vi "IL Chain Handle Last Ack.vi"(8 "error in (no error)":errorcluster, 10 "Last Ack":refnum<class "Last Ack.lvclass">, 11 "Interlock Chain in":refnum<class "Interlock Chain.lvclass">) -> (0 "error out":errorcluster, 3 "Interlock Chain out":refnum<class "Interlock Chain.lvclass">)   [LabVIEW 2015, in "Interlocks.lvlib" / "Interlock Chain.lvclass"]
uses:
  Interlock Chain.lvclass
  <vilib>/ActorFramework/LastAck/Last Ack.lvclass
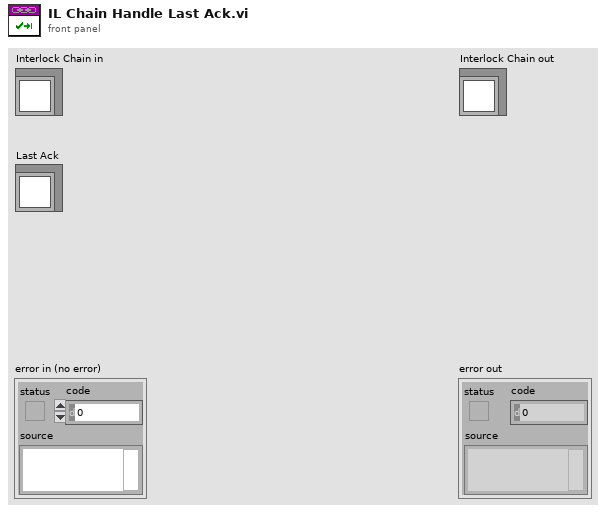
[diagram p1: front panel]
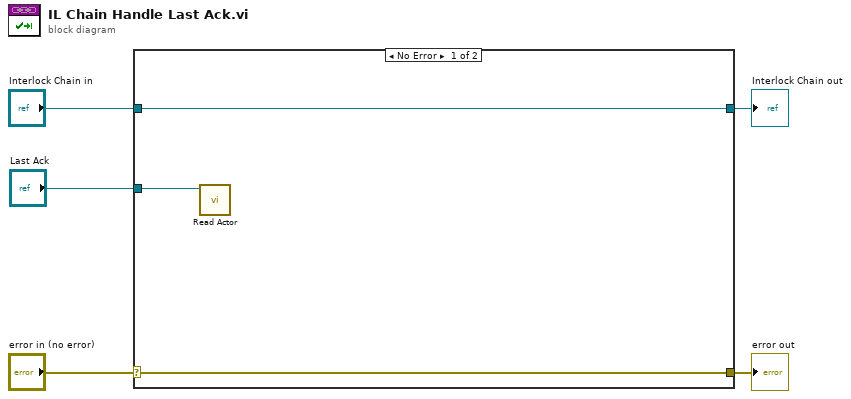
[diagram p0: block diagram]
diagram:
  n1 = case shown="No Error" "error in (no error)" {
    selector: "error in (no error)" -> [w7 w10]
    tunnel: [w7 w10] -> w4
    tunnel: [w8 w9] -> w2
    tunnel: "Interlock Chain in" -> [w8 w9]
    tunnel: "Last Ack" -> [w6 _]
    frame No Error {
      n2 = call <vilib>:"Read Actor.vi"("Last Ack"=w6) -> ()  [unwired: 10 in, 1 out]
    }
    frame Error {
    }
  }
  "error out" <- w4
  "Interlock Chain out" <- w2
